vi "ze internal querying subscriber null.vi"(8 "error in (no error)":errorcluster, 11 "this_":cluster{}) -> (0 "error out":errorcluster, 3 "this_ out":cluster{})   [LabVIEW 2021, in "zenohc.lvlib"]
doc: "ZENOHC_API void ze_internal_querying_subscriber_null(struct ze_owned_querying_subscriber_t *this_);"
uses:
  zenohc.lvlib
  zenohc.dll
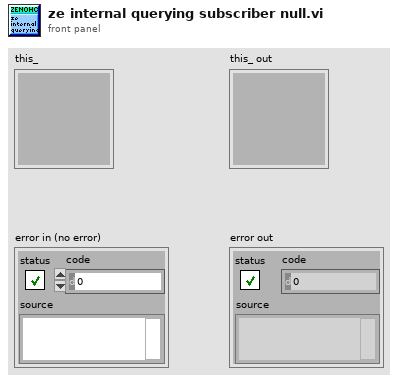
[diagram p1: front panel]
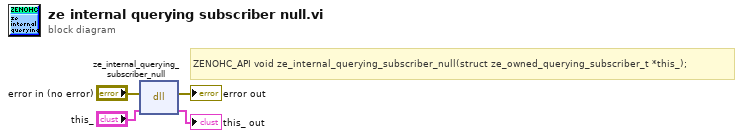
[diagram p0: block diagram]
diagram:
  # "ZENOHC_API void ze_internal_querying_subscriber_null(struct ze_owned_querying_subscriber_t *this_);"
  n1 = dll-call lib="D:/dev/zenoh_labview/zenohc/zenohc.*" fn="ze_internal_querying_subscriber_null"(error in="error in (no error)", "this_"="this_") -> (error out=→"error out":errorcluster, "this_"=→"this_ out":cluster{})  [unwired: 3 in, 1 out]
